vi "MeasureRMSJ&J (1).vi"(9 "#of Samples":dbl, 10 "Sampling Rate":dbl) -> (1 "(Vrms)":dbl format="%0.2f", 2 "Waveform Graph":dynamicdata(graph))   [LabVIEW 2015]
uses:
  <vilib>/ptbypt/NI_PtbyPt.lvlib
panel:
  in  "threshold valley":dbl format="%0.2f"
  in  "threshold peak":dbl format="%0.2f"
  out "x/y":dbl
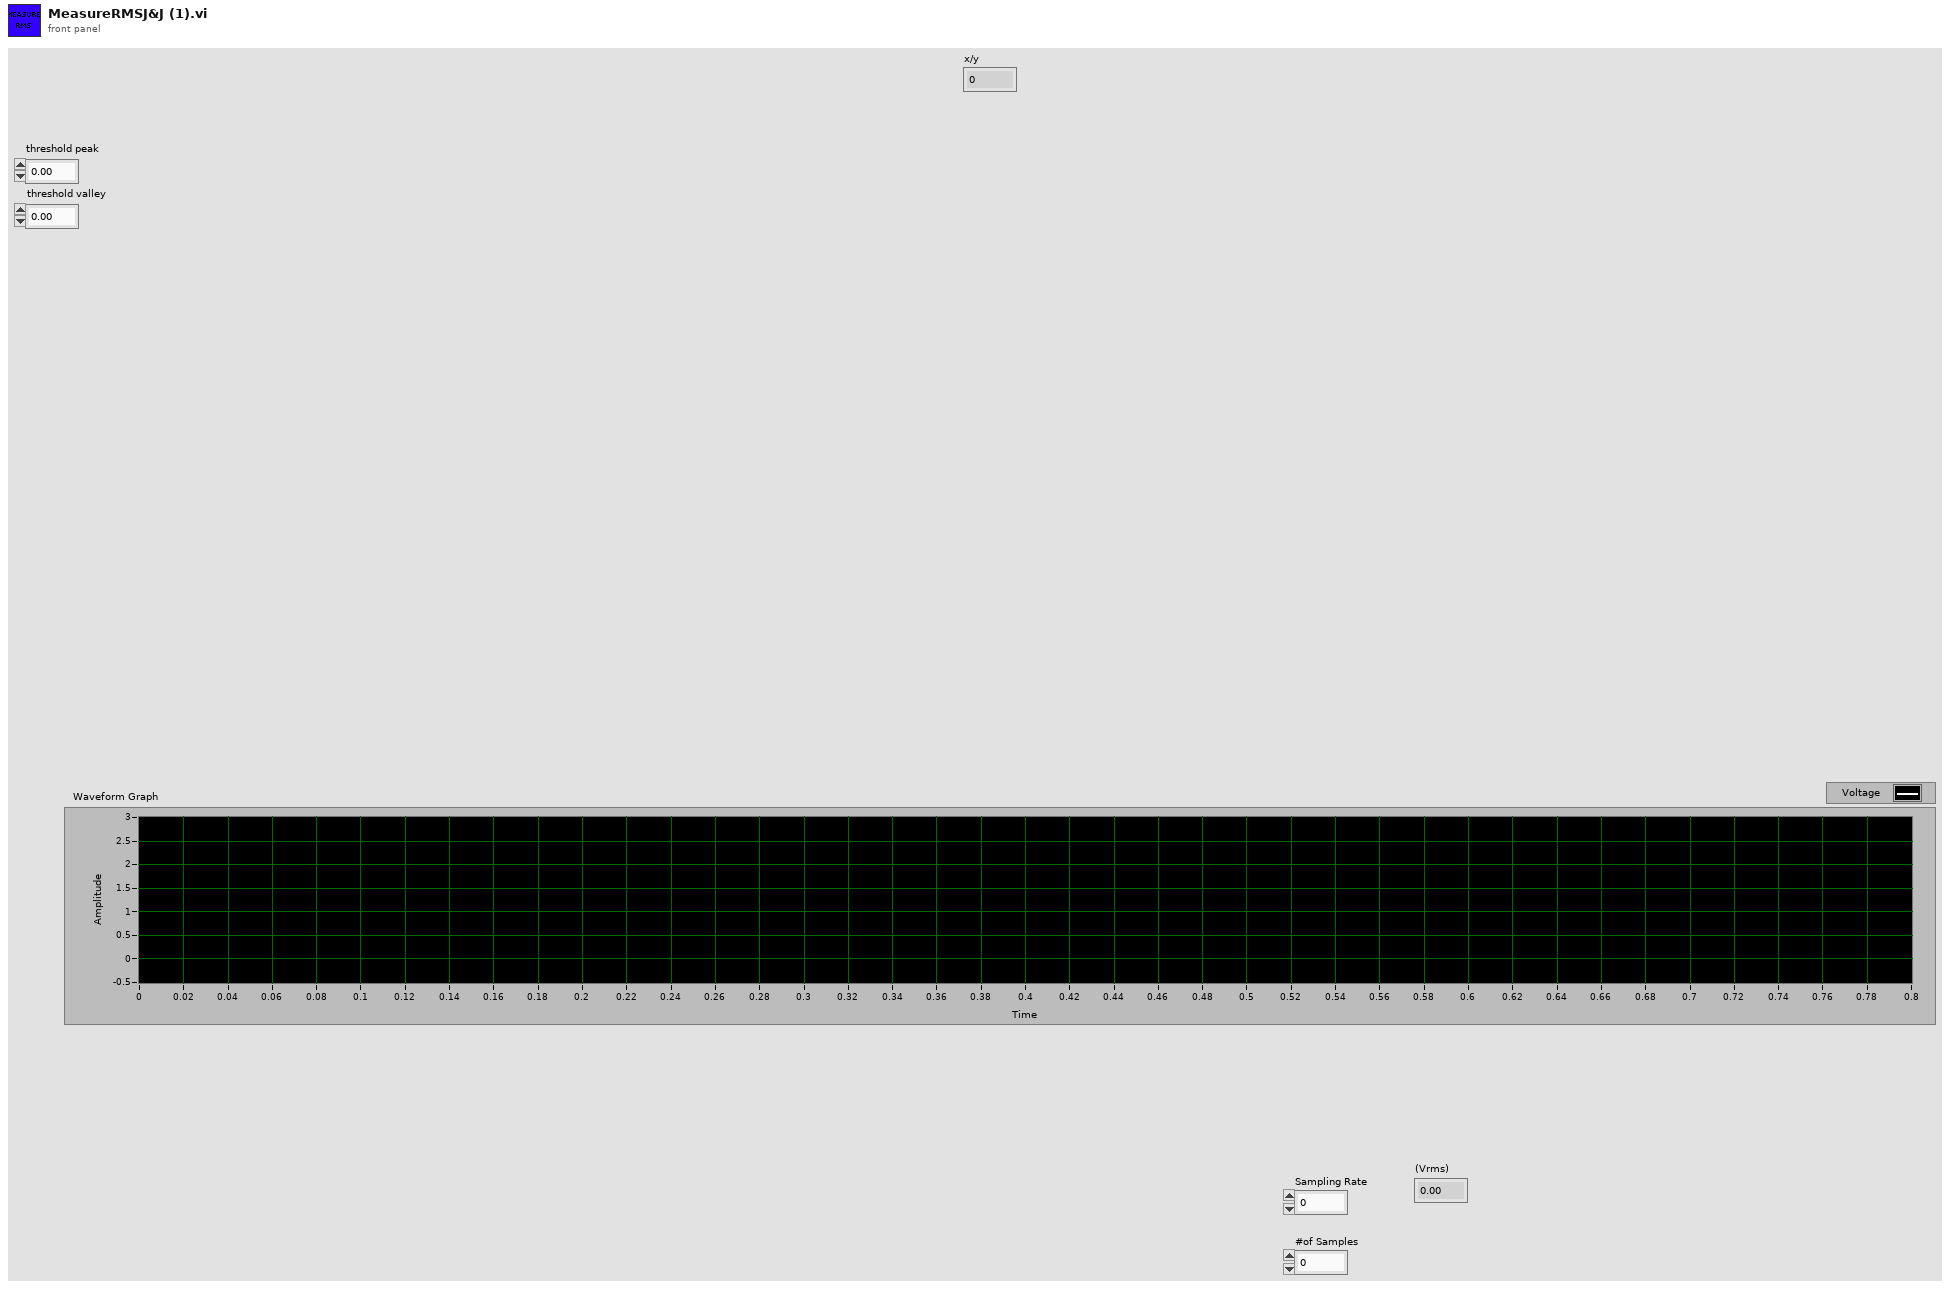
[diagram p1: front panel]
types:
  T1 = enum16{"open", "replace", "create", "open or create", "replace or create", "replace or create with confirmation"}
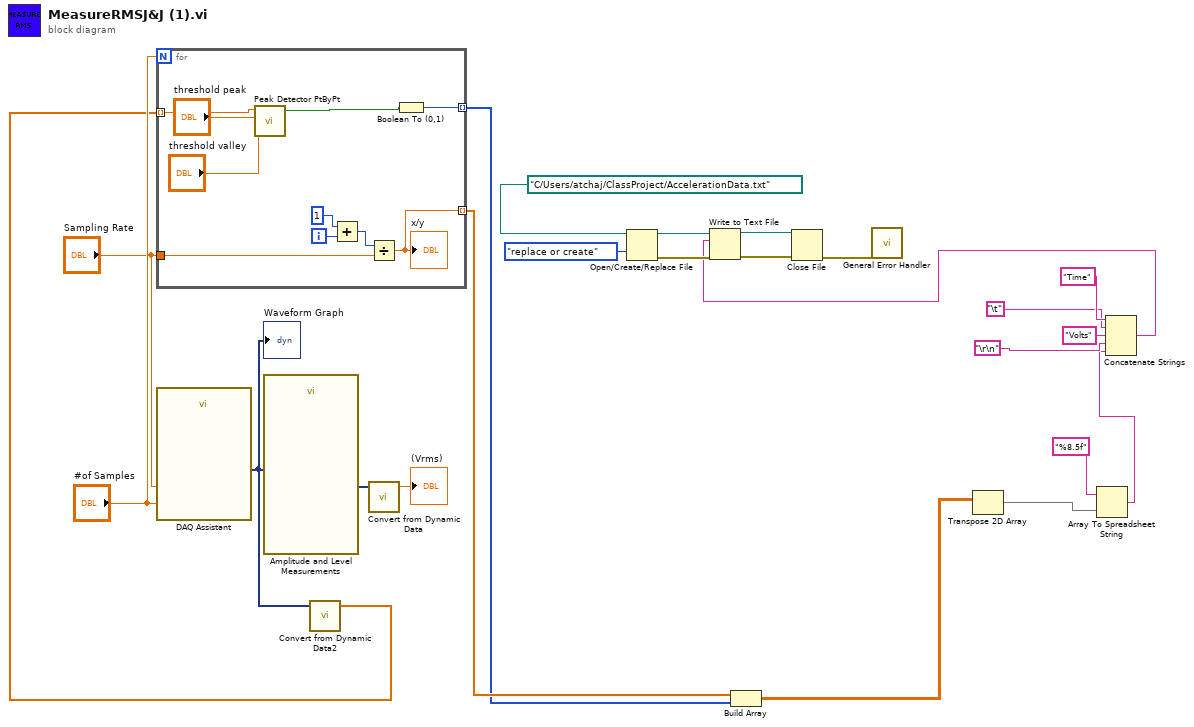
[diagram p0: block diagram]
diagram:
  n1 = call "DAQ Assistant"("rate"="Sampling Rate", "number of samples"="#of Samples") -> ("data"=w5:dynamicdata)  [unwired: 15 in, 2 out]
  "Waveform Graph" <- w5
  n2 = call "Amplitude and Level Measurements"("Signals"=w5) -> ("RMS"=w24:dynamicdata)  [unwired: 13 in, 1 out]
  n3 = call "Convert from Dynamic Data2"("Dynamic Data Type"=w5) -> ("Array"=w2:dbl[])  [unwired: 3 in]
  n4 = for {
    N: "#of Samples" -> [_]
    tunnel: "Sampling Rate" -> [w32]
    tunnel: [w30] -> w4 mode=indexing
    tunnel: w2 -> [w29] mode=indexing
    tunnel: [w25] -> w1 mode=indexing
    i -> [w34]
    n5 = call <vilib>:"Peak Detector PtByPt.vi"("x"=w29, "threshold peak"="threshold peak", "threshold valley"="threshold valley") -> ("peak"=w26:bool)  [unwired: 2 in, 2 out]
    n6 = Add(x=1, y=w34) -> (x+y=w31:i32)
    n7 = Divide(x=w31, y=w32) -> (x/y=w30:dbl)
    "x/y" <- w30
    n8 = Boolean To (0,1)(Boolean=w26) -> (0, 1=w25:i16)
  }
  n9 = call "Convert from Dynamic Data"("Dynamic Data Type"=w24) -> ("Scalar"=→"(Vrms)":dbl)  [unwired: 3 in]
  n10 = Open/Create/Replace File(file path (use dialog)=path "C:/Users/atchaj/ClassProject/AccelerationData.txt", operation (0:open)=T1."replace or create") -> (refnum out=w18:refnum<file>, error out=w19:errorcluster)  [unwired: 4 in, 1 out]
  n11 = Build Array(w4, w1) -> (w6:dbl[][])
  n12 = Transpose 2D Array(2D array=w6) -> (transposed array=w3:dbl[][])
  n13 = Array To Spreadsheet String(array=w3, 3:"%8.5f" ("format string")) -> (spreadsheet string=w10:string)  [unwired: 1 in]
  n14 = Concatenate Strings("Time" ("string"), "\t", "Volts" ("string"), "\r\n", w10) -> (w9:string)
  n15 = Write to Text File(file (use dialog)=w18, text=w9, error in=w19) -> (refnum out=w17:refnum<file>, error out=w20:errorcluster)  [unwired: 1 in, 1 out]
  n16 = Close File(refnum=w17, error in=w20) -> (error out=w21:errorcluster)  [unwired: 1 out]
  n17 = call <vilib>:"General Error Handler.vi"("error in (no error)"=w21) -> ()  [unwired: 10 in, 5 out]
